vi "WebcamReadandOverlay.vi"(8 "SurreyPath?":bool, 9 "BaseName":string, 10 "BasePathToSaveTo":path, 11 "WebcamFilePath":path) -> (1 "picturePaths":path[](array[path]), 7 "OverlayText":string)   [LabVIEW 2022 SP3]
uses:
  <vilib>/Utility/config.llb/NI_LVConfig.lvlib
  <vilib>/Utility/config.llb/Write Key (String).vi
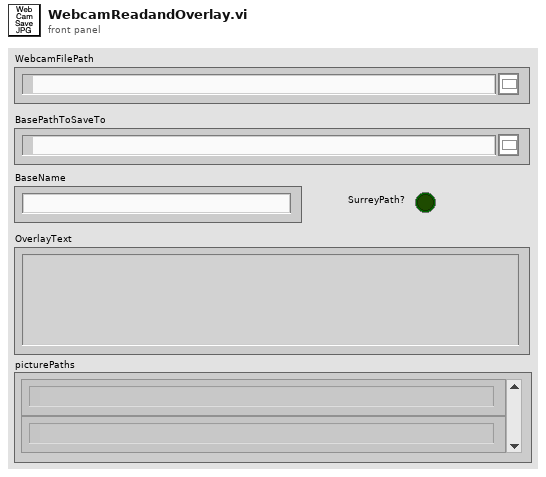
[diagram p1: front panel]
types:
  T1 = typedef "camCluster.ctl" = cluster{"cam":string, "URL":string, "ADAMspecs":cluster{"channel":string, "labelText":string, "formatString":string}[]}
  T2 = typedef "NI_LVConfig.lvlib/Config Data RefNum.ctl" = refnum<k1>
  T3 = cluster{"channel":string, "labelText":string, "formatString":string}[]
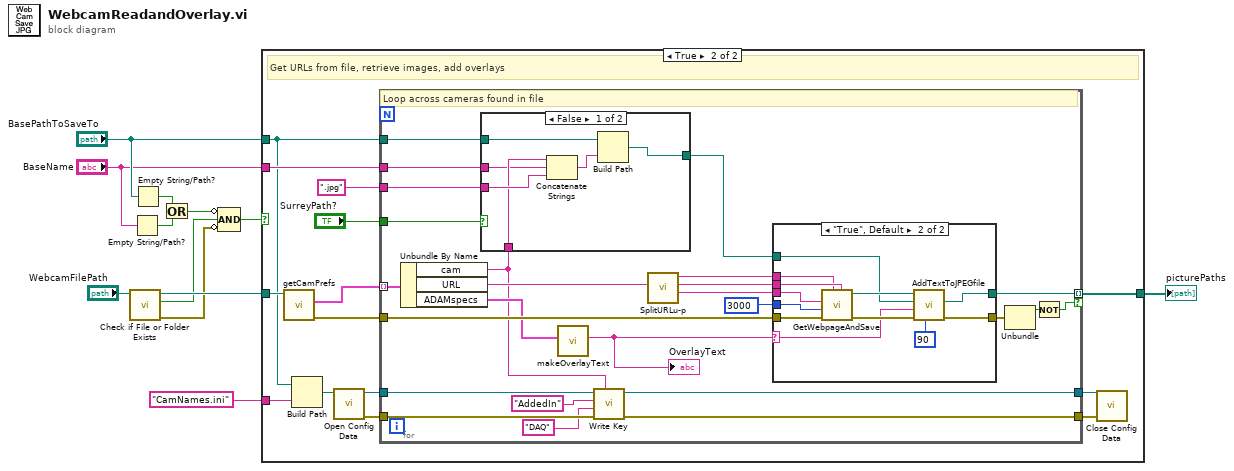
[diagram p0: block diagram]
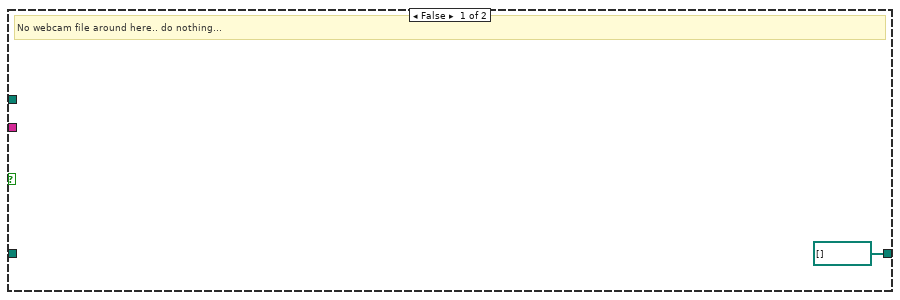
[diagram p2: hidden frame]
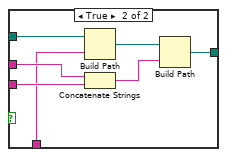
[diagram p3: hidden frame]
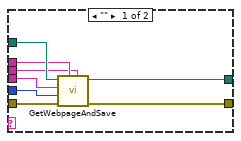
[diagram p4: hidden frame]
diagram:
  n1 = call <vilib>:"Check if File or Folder Exists.vi"("path"="WebcamFilePath") -> ("error out"=w2:errorcluster, "file or folder exists?"=w10:bool, "dup path"=w11:path)  [unwired: 8 in]
  n2 = Empty String/Path?(string/path="BaseName") -> (empty?=w6:bool)
  n3 = Empty String/Path?(string/path="BasePathToSaveTo") -> (empty?=w5:bool)
  n4 = Or(x=w5, y=w6) -> (x .or. y?=w3:bool)
  n5 = Compound Arithmetic op=AND(invert w3, w10, invert w2) -> (w4:bool)
  n6 = case shown="True" w4 {
    tunnel: w11 -> [_ w21]
    tunnel: [path[] [] w23] -> w9
    tunnel: "BaseName" -> [_ w22]
    tunnel: "BasePathToSaveTo" -> [_ w14]
    tunnel: "CamNames.ini" -> [_ w15]
    frame False {
      # "No webcam file around here.. do nothing..."
    }
    frame True {
      # "Get URLs from file, retrieve images, add overlays"
      n7 = call "getCamPrefs.vi"("INIfilePath"=w21) -> ("Error Out"=w25:errorcluster, "Array"=w27:T1[])  [unwired: 9 in]
      n8 = Build Path(base path=w14, name or relative path=w15) -> (appended path=w16:path)
      n9 = call <vilib>:"Open Config Data.vi"("configuration file path"=w16) -> ("error out"=w20:errorcluster, "refnum"=w18:T2)  [unwired: 8 in, 1 out]
      n10 = for {
        tunnel: w14 -> [w52]
        tunnel: w27 -> [w47] mode=indexing
        tunnel: ".jpg" -> [w51]
        tunnel: w22 -> [w46]
        tunnel: w25 -> [w50]
        tunnel: "SurreyPath?" -> [w45]
        tunnel: [w41] -> w23 mode=indexing if=w35
        tunnel: w20 -> [w34]
        tunnel: [w33] -> w19
        tunnel: w18 -> [w32]
        tunnel: [w31] -> w17
        # "Loop across cameras found in file"
        n11 = Unbundle By Name(w47) -> ("cam"=w30:string, "URL"=w40:string, "ADAMspecs"=w39:T3)
        n12 = case shown="False" w45 {
          tunnel: w52 -> [w58 w61]
          tunnel: w51 -> [w56 w64]
          tunnel: [w55 w63] -> w49
          tunnel: w30 -> [w54 w60]
          tunnel: w46 -> [w53 w62]
          frame False {
            n13 = Concatenate Strings(w54, w53, w56) -> (w57:string)
            n14 = Build Path(base path=w58, name or relative path=w57) -> (appended path=w55:path)
          }
          frame True {
            n15 = Build Path(base path=w61, name or relative path=w60) -> (appended path=w59:path)
            n16 = Concatenate Strings(w62, w64) -> (w65:string)
            n17 = Build Path(base path=w59, name or relative path=w65) -> (appended path=w63:path)
          }
        }
        n18 = call "makeOverlayText.vi"("ADAMspecs"=w39) -> ("OverlayText"=w38:string)  [unwired: 10 in]
        "OverlayText" <- w38
        n19 = call-poly <vilib>:"Write Key.vi"("section"=w30, "error in (no error)"=w34, "value"="DAQ" ("key"), "key"="AddedIn", "refnum"=w32) -> ("error out"=w33:errorcluster, "refnum out"=w31:T2)  [unwired: 4 in, 1 out]
        n20 = call "SplitURLu-p.vi"("url|u:p"=w40) -> ("URL"=w44:string, "pasword"=w42:string, "username"=w43:string)  [unwired: 8 in]
        n21 = case shown="\"True\", Default" w38 {
          selector: w38 -> [_ w76]
          tunnel: w50 -> [w73 w85]
          tunnel: w49 -> [w70 w78]
          tunnel: w44 -> [w72 w84]
          tunnel: 3000 ("timeout (ms)") -> [w71 w83]
          tunnel: w43 -> [w69 w80]
          tunnel: w42 -> [w68 w81]
          tunnel: [w67 w75] -> w41
          tunnel: [w66 w74] -> w37
          frame "" {
            n22 = call "GetWebpageAndSave.vi"("password"=w68, "username"=w69, "Error In"=w73, "timeout (ms)"=w71, "url"=w72, "pathIn"=w70) -> ("error out"=w66:errorcluster, "pathOut"=w67:path)  [unwired: 4 in]
          }
          frame "True", Default {
            n23 = call "GetWebpageAndSave.vi"("password"=w81, "username"=w80, "Error In"=w85, "timeout (ms)"=w83, "url"=w84) -> ("error out"=w82:errorcluster, "pathOut"=w79:path)  [unwired: 5 in]
            n24 = call "AddTextToJPEGfile.vi"("quality (80)"=90, "error in (no error)"=w82, "text"=w76, "savePath"=w78, "loadPath"=w79) -> ("error out"=w74:errorcluster, "finalPath"=w75:path)  [unwired: 5 in]
          }
        }
        n25 = Unbundle(w37) -> ("status"=w36:bool)  [unwired: 2 out]
        n26 = Not(x=w36) -> (.not. x?=w35:bool)
      }
      n27 = call <vilib>:"Close Config Data.vi"("error in (no error)"=w19, "refnum"=w17) -> ()  [unwired: 8 in, 2 out]
    }
  }
  "picturePaths" <- w9
